vi "RAMP_initialize_Z_ramp.vi"(4 "Symmetric":bool=TRUE, 5 "error in":errorcluster, 7 "Total range (nm)":u32, 8 "dZ (nm)":u32) -> (0 "error out":errorcluster, 1 "Total # steps":i32, 2 "Ramp":dbl[](array[numeric]), 3 "z0":dbl)   [LabVIEW 2015]
uses:
  GLOBAL/Global_MCL_piezo.vi
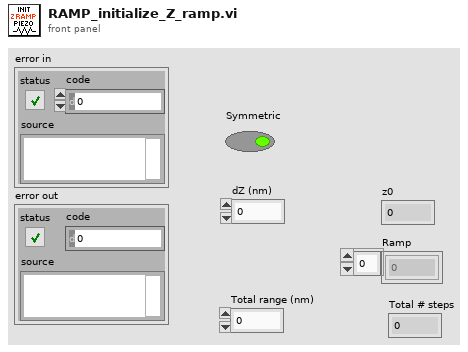
[diagram p1: front panel]
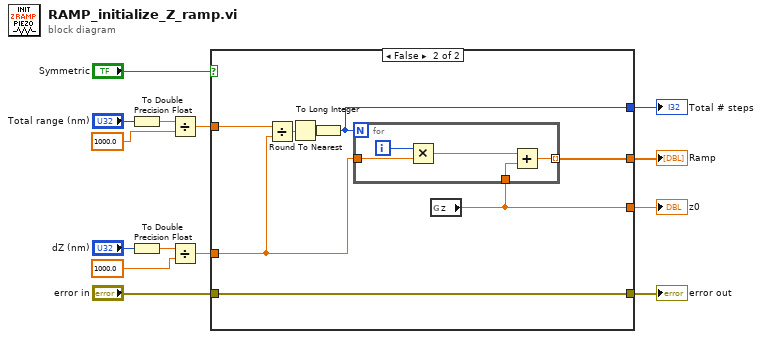
[diagram p0: block diagram]
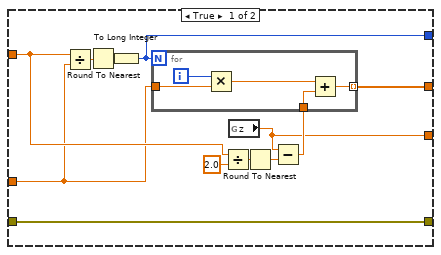
[diagram p2: hidden frame]
diagram:
  n1 = To Double Precision Float(number="Total range (nm)") -> (double precision float=w11:dbl)
  n2 = To Double Precision Float(number="dZ (nm)") -> (double precision float=w10:dbl)
  n3 = Divide(x=w11, y=1000.0) -> (x/y=w9:dbl)
  n4 = Divide(x=w10, y=1000.0) -> (x/y=w5:dbl)
  n5 = case shown="False" "Symmetric" {
    tunnel: w9 -> [w20 w37]
    tunnel: [w15 w32] -> w7
    tunnel: [w19 w36] -> w6
    tunnel: w5 -> [w18 w35]
    tunnel: [w17 w34] -> w4
    tunnel: "error in" -> [w16 w33]
    tunnel: [w16 w33] -> w1
    frame True {
      n6 = Divide(x=w20, y=w18) -> (x/y=w26:dbl)
      n7 = Round To Nearest(number=w26) -> (nearest integer value=w25:dbl)
      n8 = To Long Integer(number=w25) -> (32bit integer=w15:i32)
      n9 = Divide(x=w20, y=2.0) -> (x/y=w23:dbl)
      n10 = global read "Global_MCL_piezo.vi" "z"() -> (w17:dbl)
      n11 = Round To Nearest(number=w23) -> (nearest integer value=w21:dbl)
      n12 = Subtract(x=w17, y=w21) -> (x-y=w22:dbl)
      n13 = for {
        N: w15 -> [_]
        tunnel: w18 -> [w30]
        tunnel: w22 -> [w28]
        tunnel: [w27] -> w19 mode=indexing
        i -> [w31]
        n14 = Multiply(x=w31, y=w30) -> (x*y=w29:dbl)
        n15 = Add(x=w29, y=w28) -> (x+y=w27:dbl)
      }
    }
    frame False {
      n16 = Divide(x=w37, y=w35) -> (x/y=w39:dbl)
      n17 = Round To Nearest(number=w39) -> (nearest integer value=w38:dbl)
      n18 = To Long Integer(number=w38) -> (32bit integer=w32:i32)
      n19 = global read "Global_MCL_piezo.vi" "z"() -> (w34:dbl)
      n20 = for {
        N: w32 -> [_]
        tunnel: w35 -> [w43]
        tunnel: w34 -> [w41]
        tunnel: [w40] -> w36 mode=indexing
        i -> [w44]
        n21 = Multiply(x=w44, y=w43) -> (x*y=w42:dbl)
        n22 = Add(x=w42, y=w41) -> (x+y=w40:dbl)
      }
    }
  }
  "Total # steps" <- w7
  "Ramp" <- w6
  "error out" <- w1
  "z0" <- w4
